vi "Pivot Start BAP7.vi"(11 "BrickReference in":T1) -> (3 "BrickReference out":T1)   [LabVIEW 2014]
doc: "Pivot Start BAP7\n\nRotates 180 degrees so that it enters the ring from its front end.\n\nBeverly Abadines\nPHY 350\nBAP7"
uses:
  <vilib>/NXT/Subs/LVHSConnector.ctl
  <vilib>/NXT/LegoClasses/BrickReference/BrickReference.lvclass
  <vilib>/NXT/Block Support/NXT_OutputPort.ctl
  <vilib>/NXT/NXTIO Xnodes/NXTIONodeSubVIs/NXTMoveMotors.vi
  <vilib>/NXT/NXTIO Xnodes/AddressXNode/NXTIOAddress.xnode
  <vilib>/NXT/NXTIO Xnodes/NXTIOXNode/NXTIO.xnode
panel:
  # "Pivot Start"
  # "Beverly Abadines\nPhys 350\nP7"
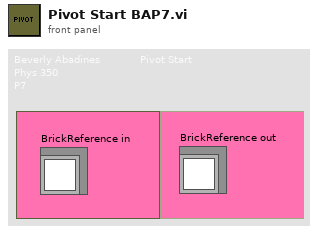
[diagram p1: front panel]
types:
  T1 = typedef "LVHSConnector.ctl" = refnum<class "BrickReference.lvclass">
  T2 = typedef "NXT_OutputPort.ctl" = u8
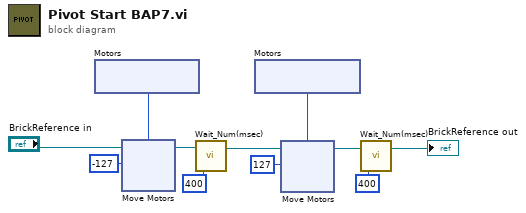
[diagram p0: block diagram]
diagram:
  n1 = xnode "Motors"() -> ("Motor"=w1:T2)
  n2 = xnode "Move Motors"("Power/Speed 1"=i8 -127, "Motors"=w1, "NXT/EV3"="BrickReference in") -> ("NXT/EV3"=w5:T1)
  n3 = call <vilib>:"Wait_Num(msec).vi"("Time (100 msec)"=u32 400, "NXT/EV3"=w5) -> ("NXT/EV3"=w6:T1)  [unwired: 2 in]
  n4 = xnode "Motors"() -> ("Motor"=w2:T2)
  n5 = xnode "Move Motors"("Power/Speed 1"=i8 127, "Motors"=w2, "NXT/EV3"=w6) -> ("NXT/EV3"=w7:T1)
  n6 = call <vilib>:"Wait_Num(msec).vi"("Time (100 msec)"=u32 400, "NXT/EV3"=w7) -> ("NXT/EV3"=→"BrickReference out":T1)  [unwired: 2 in]
